vi "Reset_Enable_Configuration_Payload.vi"(11 "identifier selection in":u8 format="%x") -> (1 "Reset errors command":T1 {"payload" format="%x"; "timestamp" format="%<%I:%M:%S%8u %p\n%x>T"; "identifier" format="%x"}, 2 "Enable motor command":T1 {"payload" format="%x"; "timestamp" format="%<%I:%M:%S%8u %p\n%x>T"; "identifier" format="%x"})   [LabVIEW 2015]
uses:
  <vilib>/Stratom, Inc/X-CAN for myRIO (API)/X-CAN Class/Type Definitions/CANFrame.ctl
  <vilib>/Stratom, Inc/X-CAN for myRIO (API)/X-CAN Class/X-CAN.lvclass
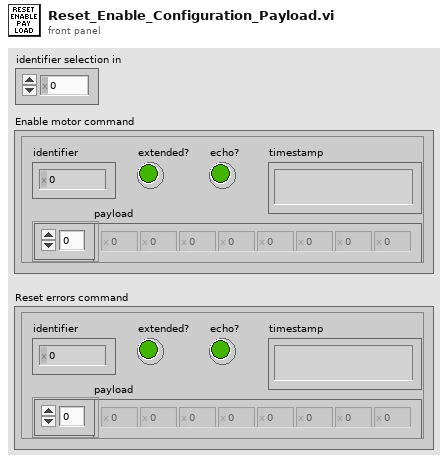
[diagram p1: front panel]
types:
  T1 = typedef "X-CAN.lvclass/CANFrame.ctl" = cluster{"identifier":u32, "extended?":bool, "echo?":bool, "payload":u8[], "timestamp":timestamp}
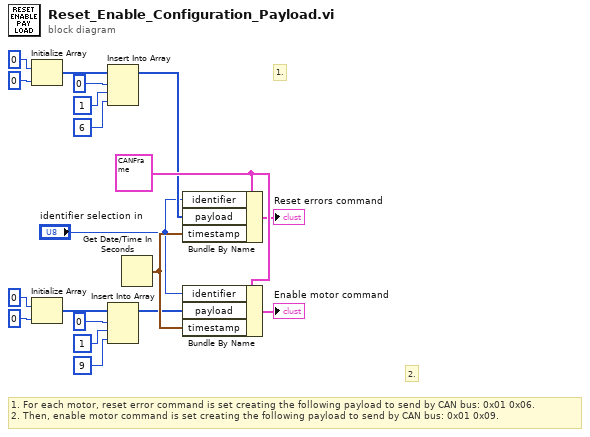
[diagram p0: block diagram]
diagram:
  w18 = T1 {"identifier"=0, "extended?"=FALSE, "echo?"=FALSE, "payload"=[], "timestamp"=timestamp(0 s since 1904-01-01)} ("CAN Frame")
  # "2."
  # "1."
  # "1. For each motor, reset error command is set creating the following payload to send by CAN bus: 0x01 0x06.\n2. Then, enable motor command is set creating the following payload to send by CAN bus: 0x01 0x09."
  n1 = Initialize Array(u16 0 ("element"), 0 ("dimension size")) -> (w7:u16[])
  n2 = Initialize Array(u16 0 ("element"), 0 ("dimension size")) -> (w15:u16[])
  n3 = Insert Into Array(array=w7, index=0, new element #1=u8 1 ("new element/subarray"), new element #2=u8 6 ("new element/subarray")) -> (w3:u16[])
  n4 = Insert Into Array(array=w15, index=0, new element #1=u8 1 ("new element/subarray"), new element #2=u8 9 ("new element/subarray")) -> (w11:u16[])
  n5 = Get Date/Time In Seconds() -> (seconds since 1Jan1904=w19:timestamp)
  n6 = Bundle By Name(cluster=w18, "identifier"="identifier selection in", "payload"=w3, "timestamp"=w19) -> (→"Reset errors command":T1)
  n7 = Bundle By Name(cluster=w18, "identifier"="identifier selection in", "payload"=w11, "timestamp"=w19) -> (→"Enable motor command":T1)
